vi "3. State Machine Based Traffic Light Simulator.vi"() -> ()   [LabVIEW 2018]
panel:
  in  "stop":bool
  out "Yellow":bool
  out "Green":bool
  out "Red":bool
  out "Traffic Lights Picture":picture
  # "Traffic Light Graphic Vector by Vecteezy\n(https://www.vecteezy.com/free-vector/graphic)"
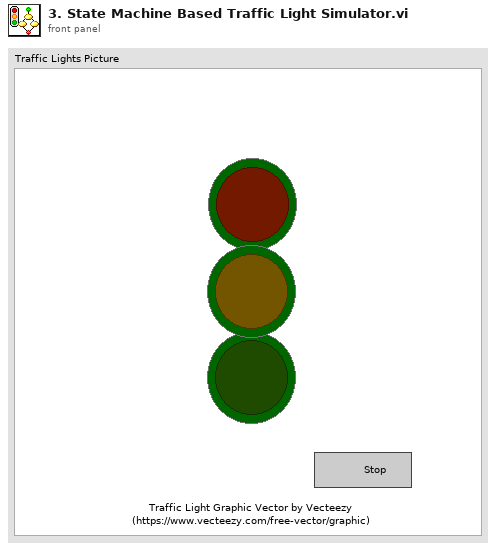
[diagram p1: front panel]
types:
  T1 = cluster{"Wait Before Red":u32, "Wait Before Yellow":u32, "Wait Before Green":u32}
  T2 = enum16{"Initialize", "Red", "Yellow", "Green", "Wait Before Red", "Wait Before Yellow", "Wait Before Green", "Stop"}
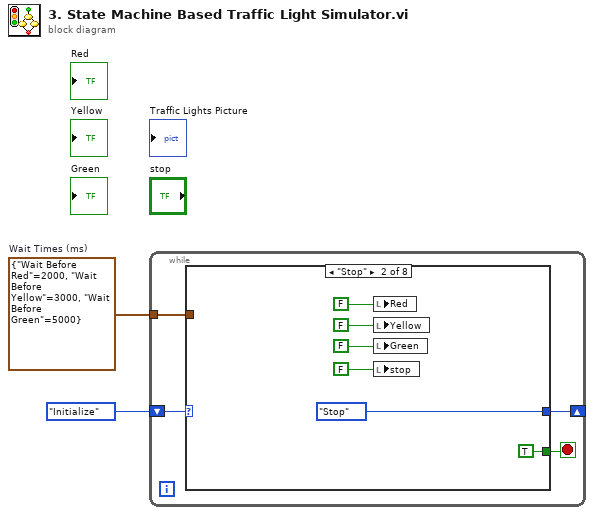
[diagram p0: block diagram]
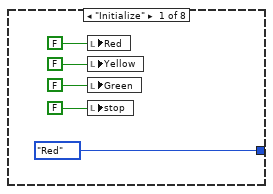
[diagram p2: hidden frame]
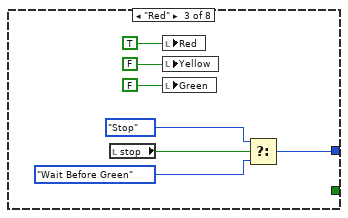
[diagram p3: hidden frame]
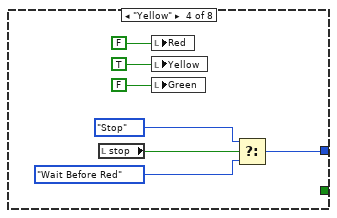
[diagram p4: hidden frame]
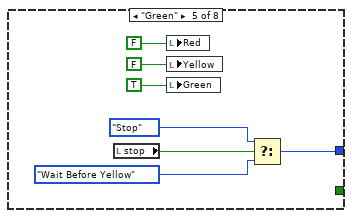
[diagram p5: hidden frame]
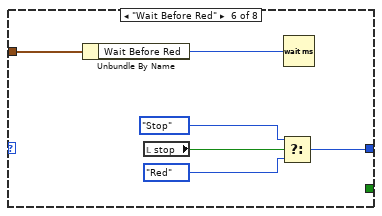
[diagram p6: hidden frame]
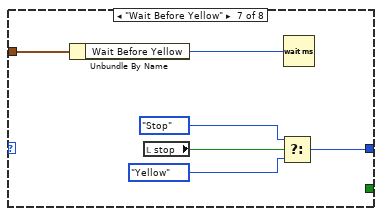
[diagram p7: hidden frame]
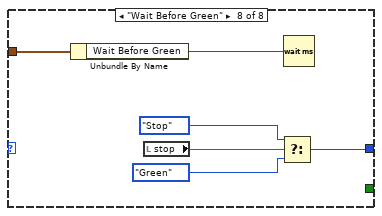
[diagram p8: hidden frame]
diagram:
  w1 = T1 {"Wait Before Red"=2000, "Wait Before Yellow"=3000, "Wait Before Green"=5000}  # Wait Times (ms)
  n1 = while {
    shift-right: [w5] -> _
    shift-left: T2."Initialize" -> [w6]
    tunnel: w1 -> [w4]
    stop <- w3 stop-if-true
    n2 = case shown="\"Stop\"" w6 {
      tunnel: [T2."Red" T2."Stop" w22 w29 w36 w43 w49 w55] -> w5
      tunnel: w4 -> [_ _ _ _ _ w40 w46 w52]
      tunnel: [_ TRUE _ _ _ _ _ _] -> w3
      frame "Initialize" {
        n3 = local write "Red"(FALSE ("Red")) -> ()
        n4 = local write "Yellow"(FALSE ("Red")) -> ()
        n5 = local write "Green"(FALSE ("Red")) -> ()
        n6 = local write "stop"(FALSE ("stop")) -> ()
      }
      frame "Stop" {
        n7 = local write "Red"(FALSE ("Red")) -> ()
        n8 = local write "Yellow"(FALSE ("Red")) -> ()
        n9 = local write "Green"(FALSE ("Red")) -> ()
        n10 = local write "stop"(FALSE ("stop")) -> ()
      }
      frame "Red" {
        n11 = local read "stop"() -> (w23:bool)
        n12 = local write "Red"(TRUE ("Red")) -> ()
        n13 = local write "Yellow"(FALSE ("Red")) -> ()
        n14 = local write "Green"(FALSE ("Red")) -> ()
        n15 = Select(t=T2."Stop", s=w23, f=T2."Wait Before Green") -> (s? t:f=w22:T2)
      }
      frame "Yellow" {
        n16 = local read "stop"() -> (w30:bool)
        n17 = local write "Red"(FALSE ("Red")) -> ()
        n18 = local write "Yellow"(TRUE ("Red")) -> ()
        n19 = local write "Green"(FALSE ("Red")) -> ()
        n20 = Select(t=T2."Stop", s=w30, f=T2."Wait Before Red") -> (s? t:f=w29:T2)
      }
      frame "Green" {
        n21 = local read "stop"() -> (w37:bool)
        n22 = local write "Red"(FALSE ("Red")) -> ()
        n23 = local write "Yellow"(FALSE ("Red")) -> ()
        n24 = local write "Green"(TRUE ("Red")) -> ()
        n25 = Select(t=T2."Stop", s=w37, f=T2."Wait Before Yellow") -> (s? t:f=w36:T2)
      }
      frame "Wait Before Red" {
        n26 = Unbundle By Name(w40) -> ("Wait Before Red"=w39:u32)
        n27 = local read "stop"() -> (w44:bool)
        n28 = Select(t=T2."Stop", s=w44, f=T2."Red") -> (s? t:f=w43:T2)
        n29 = Wait (ms)(milliseconds to wait=w39) -> ()  [unwired: 1 out]
      }
      frame "Wait Before Yellow" {
        n30 = Unbundle By Name(w46) -> ("Wait Before Yellow"=w45:u32)
        n31 = local read "stop"() -> (w50:bool)
        n32 = Select(t=T2."Stop", s=w50, f=T2."Yellow") -> (s? t:f=w49:T2)
        n33 = Wait (ms)(milliseconds to wait=w45) -> ()  [unwired: 1 out]
      }
      frame "Wait Before Green" {
        n34 = Unbundle By Name(w52) -> ("Wait Before Green"=w51:u32)
        n35 = local read "stop"() -> (w56:bool)
        n36 = Select(t=T2."Stop", s=w56, f=T2."Green") -> (s? t:f=w55:T2)
        n37 = Wait (ms)(milliseconds to wait=w51) -> ()  [unwired: 1 out]
      }
    }
  }
